vi "Switch Button Click Counter - v01.vi"(2 "Numeric":i32, 3 "Klik":bool) -> (0 "Output":bool, 1 "Klik Counter":i32)   [LabVIEW 2013]
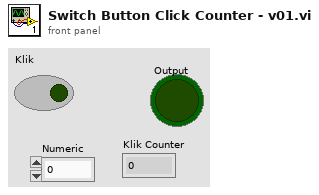
[diagram p1: front panel]
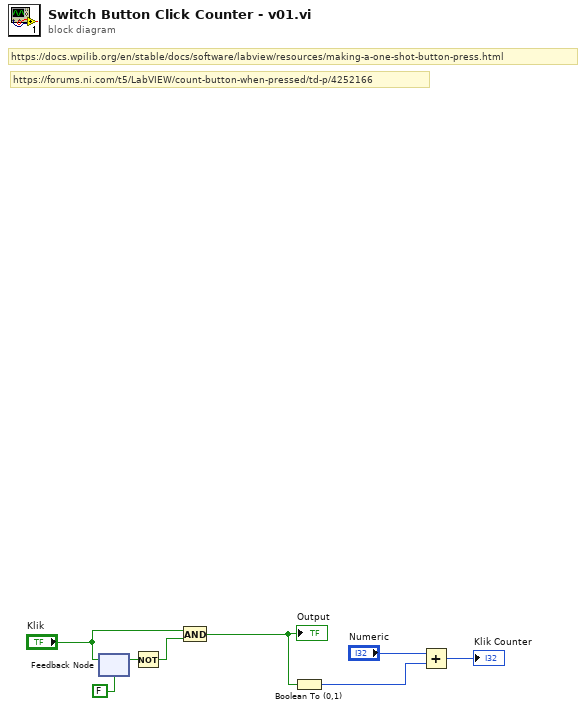
[diagram p0: block diagram]
diagram:
  # "https://forums.ni.com/t5/LabVIEW/count-button-when-pressed/td-p/4252166"
  # "https://docs.wpilib.org/en/stable/docs/software/labview/resources/making-a-one-shot-button-press.html"
  n1 = feedback #1(FALSE ("Boolean")) -> (w7:bool)
  n2 = feedback-in #1("Klik") -> ()
  n3 = Not(x=w7) -> (.not. x?=w5:bool)
  n4 = And(x="Klik", y=w5) -> (x .and. y?=w4:bool)
  "Output" <- w4
  n5 = Boolean To (0,1)(Boolean=w4) -> (0, 1=w3:i16)
  n6 = Add(x="Numeric", y=w3) -> (x+y=→"Klik Counter":i32)
